vi "Default Settings.vi"(8 "error in (no error)":errorcluster, 11 "C4 Dispense in 2":refnum<class "Dispense Offset.lvclass">) -> (0 "error out":errorcluster, 3 "C4 Dispense out 2":refnum<class "Dispense Offset.lvclass">)   [LabVIEW 2019, in "Dispense Offset.lvclass"]
uses:
  Dispense Offset.lvclass
  C:/Users/HEP/Documents/Aerotech gantry/UCSB-Gantry-master-main/V5/Classes/Routine/Dispense/CAD Dispense/CAD Dispense.lvclass
  C:/Users/HEP/Documents/Aerotech gantry/UCSB-Gantry-master-main/V5/Classes/Routine/Dispense/Dispense.lvclass
  CAD Dispense/CAD Dispense.lvclass/CAD Dispense.ctl
  CAD Dispense/Read Glue Speed.vi
  CAD Dispense/Read Move Speed.vi
  CAD Dispense/CAD Dispense.lvclass
  Dispense.lvclass
panel:
  # "This Routine does not Accept Settings"
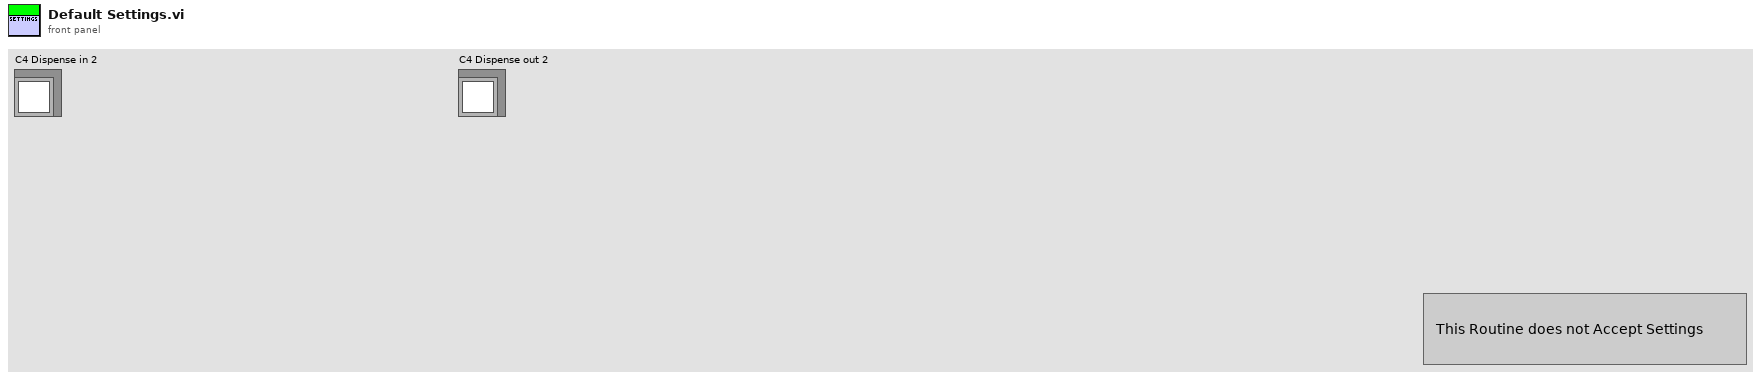
[diagram p1: front panel]
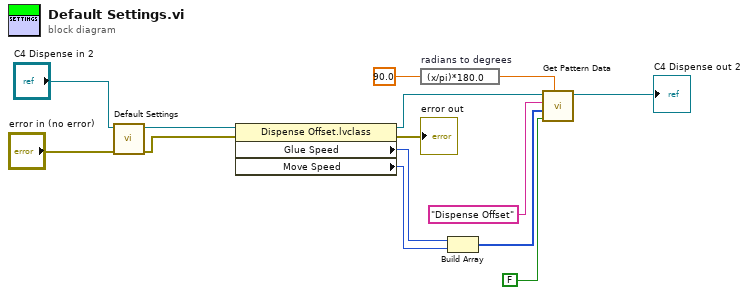
[diagram p0: block diagram]
diagram:
  n1 = call-parent "Default Settings.vi"("error in (no error)"="error in (no error)", "CAD Dispense in"="C4 Dispense in 2") -> ("error out"=w2:errorcluster, "CAD Dispense out"=w12:refnum<class "Dispense Offset.lvclass">)  [unwired: 8 in]
  n2 = property class="Dispense Offset.lvclass"(reference=w12, error in=w2) -> (reference out=w11:refnum<class "Dispense Offset.lvclass">, error out=→"error out":errorcluster, "Glue Speed"=w4:i32, "Move Speed"=w3:i32)
  n3 = expression code="(x/pi)*180.0" "radians to degrees"(90.0) -> (w7:dbl)
  n4 = Build Array(w4, w3) -> (w1:i32[])
  n5 = call "Get Pattern Data.vi"("theta"=w7, "Iterative?"=FALSE, "File Name"=w1, "Folder Name"="Dispense Offset", "Dispense.lvclass"=w11) -> ("Dispense Out"=→"C4 Dispense out 2":refnum<class "Dispense Offset.lvclass">)  [unwired: 6 in]
